vi "SetVMinVStart.vi"(0 "handle in":i32, 1 "UnitAddress(0)":u16, 2 "MotNr(0)":u8, 5 "error in":errorcluster, 7 "VminVStart":T1={"VStart(5)"=5, "Vmin(4)"=4, "Div i (2)"=enum."2"}) -> (14 "handle out":i32, 19 "error out":errorcluster)   [LabVIEW 2014, in "Sixpack - Driver.lvlib"]
doc: "ACHTUNG: nur bei stehendem Motor ändern!\n\nVMin ist nur für die Referenzfahrt relevant. Es setzt die Geschwindigkeit, etwa beim präzisen Suchen nach dem „Anschlagpunkt“ des Referenzschalters fest. \nVStart gibt die Geschwindigkeit an mit der Fahrrampen gestartet bzw. beendet werden.\n\nDurch Einstellung eines möglichst hohen Wertes für VStart, erreicht der jeweilige Motor\nschnell die maximale Geschwindigkeit und muss diese auch erst spät vor Erreichen des Ziels abbremsen. Ein zu hoher Wert kann aber dazu führen, dass der Motor nicht anlaufen kann oder die genaue Zielposition verfehlt.\n\nDiv ist der für jede Achse individuell einstellbare Schrittfrequenz-Vorteiler (siehe Manual Kapitel 3.3.1). Ein kleines Div ermöglicht hohe Schrittfrequenzen und damit maximale Achsenumdrehungen, ein großes Div hingegen erhöht die Auflösung der Geschwindigkeitsstufen und damit auch feinerer Beschleunigungsrampen. Dadurch lassen sich bei hohen Geschwindigkeiten die Zielpositionen bei Rampenfahrt präziser anfahren. \n\nCMD $13\nMotorNr (0...5)\nVMin (0..511): Minimalgeschwindigkeit für Referenzfahrt Bei Übergabe von 0 wird der optimale Wert für die Konfiguration berechnet.\n VMin <= 250Hz / fMikroschrittMin;\n VMin <= VStart (fMikroschrittMin ist die Mikroschrittfrequenz bei Geschwindigkeit 1)\nVStart (1..511): Startgeschwindigkeit bei Rampenfahrt. Zulässiger Maximalwert ist abhängig von Div:\n Div = 3: 0 < VStart < 512\n Div = 2: 0 < VStart < 256\n Div = 1: 0 < VStart < 128\n Div = 0: 0 < VStart < 64s\nDiv (0..3): s. Berechnung der Schrittfrequenz (Default: Div =2)"
uses:
  Sixpack - Driver.lvlib
  VStartVmin.ctl
  DLL/PackDLL.dll
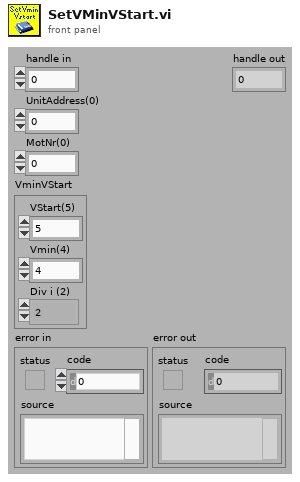
[diagram p1: front panel]
types:
  T1 = typedef "Sixpack - Driver.lvlib/VStartVmin.ctl" = cluster{"VStart(5)":u16, "Vmin(4)":u16, "Div i (2)":enum8{"0", "1", "2", "3"}}
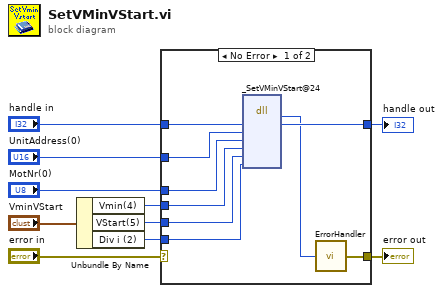
[diagram p0: block diagram]
diagram:
  n1 = Unbundle By Name("VminVStart") -> ("Vmin(4)"=w4:u16, "VStart(5)"=w3:u16, "Div i (2)"=w1:enum8{"0", "1", "2", "3"})
  n2 = case shown="No Error" "error in" {
    selector: "error in" -> [_ w20]
    tunnel: "handle in" -> [w19 w21]
    tunnel: [w18 w21] -> w9
    tunnel: "UnitAddress(0)" -> [w17 _]
    tunnel: "MotNr(0)" -> [w16 _]
    tunnel: w4 -> [w15 _]
    tunnel: w3 -> [w14 _]
    tunnel: w1 -> [w13 _]
    tunnel: [w11 w20] -> w6
    frame No Error {
      n3 = dll-call lib="D:/CS-Source/LV2014/GPL/instr.lib/SixPack/PackDLL/DLL/PackDLL.dll" fn="_SetVMinVStart@24" label="SetVMinVStart"("HANDLE"=w19, "UnitAddress"=w17, "MotNr"=w16, "VMin"=w15, "VStart"=w14, "Div"=w13) -> ("BOOLEAN"=w12:i8, "HANDLE"=w18:i32)  [unwired: 8 in, 2 out]
      n4 = call "ErrorHandler.vi"("BOOLEAN"=w12) -> ("error out"=w11:errorcluster)
    }
    frame Error {
    }
  }
  "handle out" <- w9
  "error out" <- w6
